vi "Module Init.vi"(8 "error in (no error)":errorcluster, 11 "DAQmxAO in":refnum<class "DAQmxAO.lvclass">) -> (0 "error out":errorcluster, 3 "DAQmxAO out":refnum<class "DAQmxAO.lvclass">)   [LabVIEW 2023, in "VolatusDAQ.lvlib" / "DAQmxAO.lvclass"]
uses:
  DAQmxAO.lvclass
  VolatusData/DataProc Options.ctl
  DAQmxAO.lvclass/DAQmxAO.ctl
  Volatus/Module/Module.lvclass/Module.ctl
  Volatus/MessageQ/MessageQ.lvclass/MessageQ.ctl
  Volatus/Module/Self Q.vi
  Volatus/MessageQ/Send.vi
  VolatusDAQ.lvlib
  VolatusData/Data Processor Module/Data Processor Module.lvclass
  Volatus/Module/Module.lvclass
  C:/dev/volatus/mts-volatus-super/libs/lv-volatus/Volatus/Module/Module.lvclass
  C:/dev/volatus/mts-volatus-super/libs/lv-volatus/VolatusDAQ/DAQmxAO/DAQmxAO.lvclass
  VolatusData/VolatusData.lvlib
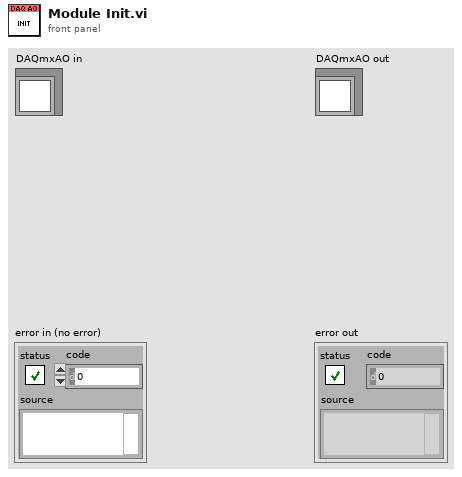
[diagram p1: front panel]
types:
  T1 = typedef "VolatusData.lvlib/DataProc Options.ctl" = cluster{"Ignore Scaling":bool}
  T2 = typedef "VolatusDAQConfig.lvlib/Sampling Config.ctl" = cluster{"Rate":dbl, "Chunk Size":i32}
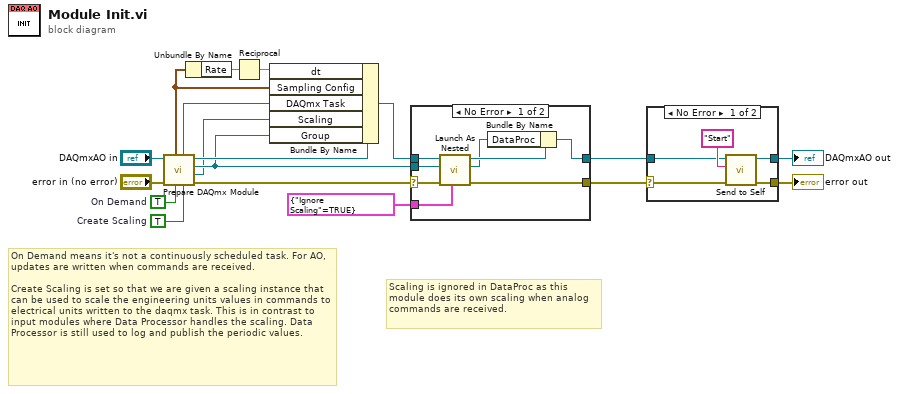
[diagram p0: block diagram]
diagram:
  w5 = TRUE  # On Demand
  w6 = TRUE  # Create Scaling
  # "Scaling is ignored in DataProc as this module does its own scaling when analog commands are received."
  # "On Demand means it's not a continuously scheduled task. For AO, updates are written when commands are received.\n\nCreate Scaling is set so that we are given a scaling instance that can be used to scale the engineering units values in commands to electrical units written to the daqmx task. This is in contrast to input modules where Data Processor handles the scaling. Data Processor is still used to log and publish the periodic values."
  n1 = call "Prepare DAQmx Module.vi"("Create Scaling (F)"=w6, "On Demand (F)"=w5, "error in (no error)"="error in (no error)", "Module in"="DAQmxAO in") -> ("error out"=w14:errorcluster, "Scaling"=w9:refnum<class "Scaling.lvclass">, "Group"=w12:refnum<class "Group DBL.lvclass">, "Module out"=w16:refnum<class "DAQmxAO.lvclass">, "DAQmx Task"=w15:refnum<k21>, "Sampling Config"=w4:T2)  [unwired: 2 in]
  n2 = Unbundle By Name(w4) -> ("Rate"=w3:dbl)
  n3 = Reciprocal(x=w3) -> (1/x=w2:dbl)
  n4 = Bundle By Name(cluster=w16, "dt"=w2, "Sampling Config"=w4, "DAQmx Task"=w15, "Scaling"=w9, "Group"=w12) -> (w13:refnum<class "DAQmxAO.lvclass">)
  n5 = case shown="No Error" w14 {
    selector: w14 -> [w26 w27]
    tunnel: w13 -> [w25 w28]
    tunnel: w12 -> [w24 _]
    tunnel: [w23 w27] -> w7
    tunnel: [w20 w28] -> w8
    tunnel: T1 {"Ignore Scaling"=TRUE} ("DataProc Options") -> [w19 _]
    frame No Error {
      n6 = call "Launch As Nested.vi"("DataProc Options"=w19, "error in (no error)"=w26, "Group"=w24, "Parent in"=w25) -> ("error out"=w23:errorcluster, "MessageQ"=w21:refnum<class "MessageQ.lvclass">, "Parent out"=w22:refnum<class "DAQmxAO.lvclass">)  [unwired: 5 in]
      n7 = Bundle By Name(cluster=w22, "DataProc"=w21) -> (w20:refnum<class "DAQmxAO.lvclass">)
    }
    frame Error {
    }
  }
  n8 = case shown="No Error" w7 {
    selector: w7 -> [w29 w35]
    tunnel: [w33 w35] -> w10
    tunnel: w8 -> [w30 w34]
    tunnel: [w32 w34] -> w11
    frame No Error {
      n9 = call "Send to Self.vi"("error in (no error)"=w29, "Message ID"="Start", "Module in"=w30) -> ("error out"=w33:errorcluster, "Module out"=w32:refnum<class "DAQmxAO.lvclass">)  [unwired: 7 in]
    }
    frame Error {
    }
  }
  "error out" <- w10
  "DAQmxAO out" <- w11
